vi "Execute_Command.vi"(1 "Debug":bool, 2 "Event":cluster{string, string[], dbl[], dbl}) -> ()   [LabVIEW 2011]
doc: "This VI contains the code to execute all gas flow/relay commands, as well as miscellaneous commands such as to enable the Vacuum or the Heater."
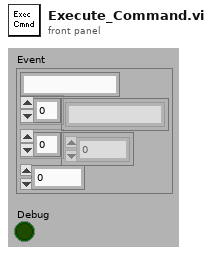
[diagram p1: front panel]
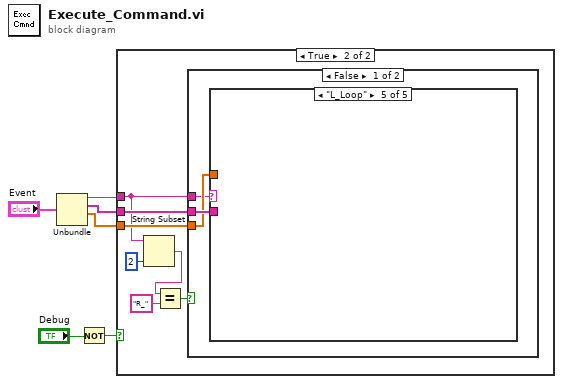
[diagram p0: block diagram]
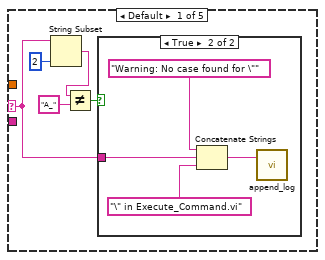
[diagram p3: hidden frame]
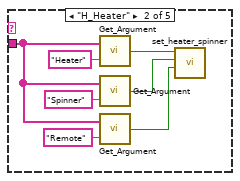
[diagram p5: hidden frame]
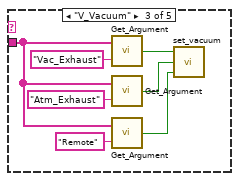
[diagram p6: hidden frame]
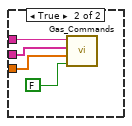
[diagram p8: hidden frame]
diagram:
  n1 = Unbundle("Event") -> (w6:string, w5:string[], w4:dbl[])  [unwired: 1 out]
  n2 = Not(x="Debug") -> (.not. x?=w3:bool)
  n3 = case shown="True" w3 {
    tunnel: w6 -> [_ w11]
    tunnel: w5 -> [_ w13]
    tunnel: w4 -> [_ w12]
    frame False {
    }
    frame True {
      n4 = String Subset(string=w11, length (rest)=2 ("length (rest)")) -> (substring=w9:string)  [unwired: 1 out]
      n5 = Equal?(x=w9, y="R_") -> (x = y?=w7:bool)
      n6 = case shown="False" w7 {
        tunnel: w13 -> [w16 w41]
        tunnel: w12 -> [w15 w42]
        tunnel: w11 -> [w14 w43]
        frame False {
          n7 = case shown="\"L_Loop\"" w14 {
            selector: w14 -> [w21 _ _ _ _]
            tunnel: w16 -> [_ w27 w34 _ _]
            tunnel: w15 -> [_ _ _ _ _]
            frame Default {
              n8 = String Subset(string=w21, length (rest)=2 ("length (rest)")) -> (substring=w18:string)  [unwired: 1 out]
              n9 = Not Equal?(x=w18, y="A_") -> (x != y?=w19:bool)
              n10 = case shown="True" w19 {
                tunnel: w21 -> [_ w22]
                frame False {
                }
                frame True {
                  n11 = Concatenate Strings("Warning: No case found for \"" ("message"), w22, "\" in Execute_Command.vi" ("string")) -> (w23:string)
                  n12 = call "append_log.vi"("New Log String"=w23) -> ()  [unwired: 1 in, 1 out]
                }
              }
            }
            frame "H_Heater" {
              n13 = call "Get_Argument.vi"("Argument"="Heater", "Argument List"=w27) -> ("Enabled"=w30:bool)
              n14 = call "Get_Argument.vi"("Argument"="Spinner", "Argument List"=w27) -> ("Enabled"=w29:bool)
              n15 = call "Get_Argument.vi"("Argument"="Remote", "Argument List"=w27) -> ("Enabled"=w26:bool)
              n16 = call "set_heater_spinner.vi"("Remote"=w26, "Spinner"=w29, "Heater"=w30) -> ()  [unwired: 7 out]
            }
            frame "V_Vacuum" {
              n17 = call "Get_Argument.vi"("Argument"="Vac_Exhaust", "Argument List"=w34) -> ("Enabled"=w37:bool)
              n18 = call "Get_Argument.vi"("Argument"="Atm_Exhaust", "Argument List"=w34) -> ("Enabled"=w36:bool)
              n19 = call "Get_Argument.vi"("Argument"="Remote", "Argument List"=w34) -> ("Enabled"=w33:bool)
              n20 = call "set_vacuum.vi"("Remote"=w33, "Atm"=w36, "Vac Exhaust"=w37) -> ()
            }
            frame "W_Wait" {
            }
            frame "L_Loop" {
            }
          }
        }
        frame True {
          n21 = call "Gas_Commands.vi"("Debug Mode"=FALSE, "Flow Array"=w42, "Argument List"=w41, "Command"=w43) -> ()  [unwired: 1 out]
        }
      }
    }
  }
